vi "StopScreen.vi"(8 "error in":errorcluster) -> (0 "error out":errorcluster)   [LabVIEW 2011]
uses:
  SubVIs/Controls/TransparencyEffectOperations.ctl
panel:
  in  "STOP":bool
  in  "CANCEL":bool
  in  "INIT":bool
  # "Do you want to Quit or Start again?"
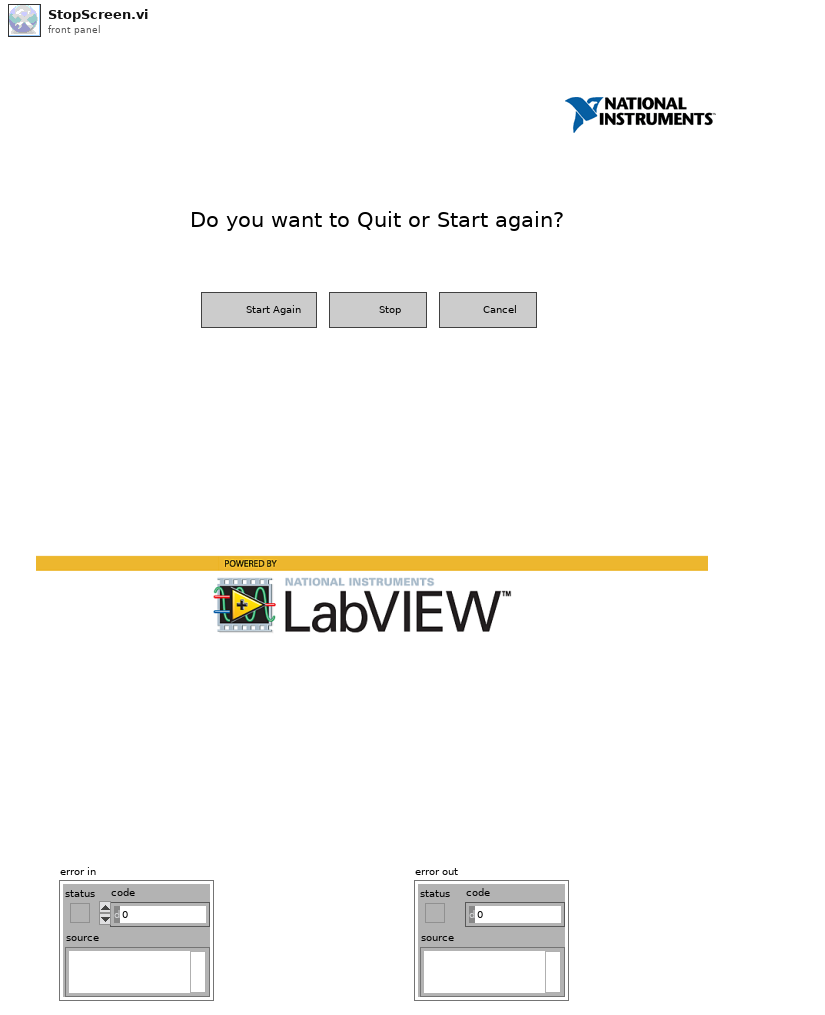
[diagram p1: front panel]
types:
  T1 = typedef "TransparencyEffectOperations.ctl" = enum16{"Show", "Hide 80%", "Hide All"}
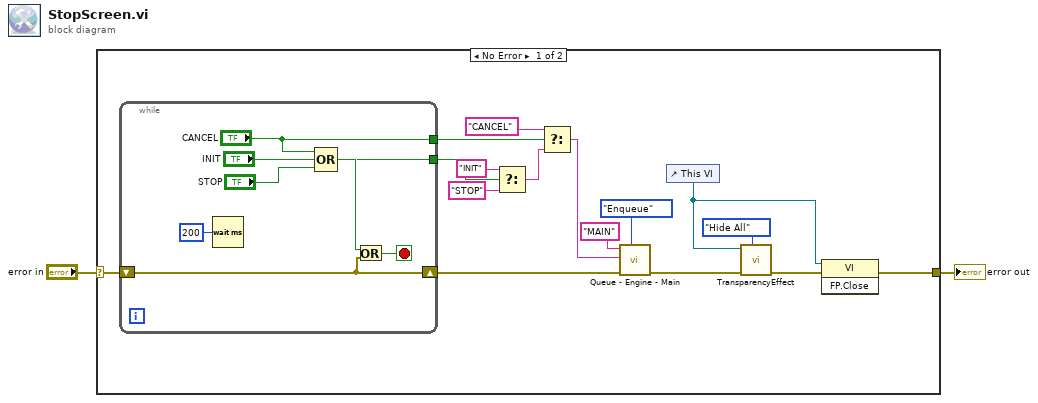
[diagram p0: block diagram]
diagram:
  n1 = case shown="No Error" "error in" {
    selector: "error in" -> [w18 w26]
    tunnel: [w3 w26] -> w2
    frame No Error {
      n2 = while {
        shift-right: [w22] -> w15
        shift-left: w18 -> [w22]
        tunnel: ["CANCEL"] -> w10
        tunnel: ["INIT"] -> w9
        stop <- w24 stop-if-true
        n3 = Wait (ms)(milliseconds to wait=u32 200) -> ()  [unwired: 1 out]
        n4 = Compound Arithmetic op=OR("CANCEL", "INIT", "STOP") -> (w25:bool)
        n5 = Or(x=w25, y=w22) -> (x .or. y?=w24:bool)
      }
      n6 = Select(t="INIT" ("Queue Name In"), s=w9, f="STOP" ("Queue Name In")) -> (s? t:f=w13:string)
      n7 = Select(t="CANCEL" ("Queue Name In"), s=w10, f=w13) -> (s? t:f=w8:string)
      n8 = call "Queue - Engine - Main.vi"("Operation"=enum16{"Enqueue", "Dequeue", "Flush", "Release"}."Enqueue", "error in"=w15, "Queue Data In"=w8, "Queue Name In"="MAIN") -> ("error out"=w6:errorcluster)  [unwired: 5 in, 2 out]
      n9 = control-ref of="This VI"() -> (w5:refnum<vi>)
      n10 = call "TransparencyEffect.vi"("Operation"=TransparencyEffectOperations."Hide All", "error in"=w6, "VI Ref in"=w5) -> ("error out"=w4:errorcluster)  [unwired: 8 in]
      n11 = invoke class="VI" method="FP.Close"(reference=w5, error in=w4) -> (error out=w3:errorcluster)  [unwired: 1 in, 2 out]
    }
    frame Error {
    }
  }
  "error out" <- w2
